vi "GDSFile_CreateFolders.vi"(1 "Path":path, 3 "Promt if folder\ndoes not exists?":bool=TRUE, 5 "error in (no error)":errorcluster) -> (13 "log error":errorcluster, 14 "PathOut":path, 15 "File permission error!":bool, 16 "Folder exists?":bool, 19 "error out":errorcluster)   [LabVIEW 2020]
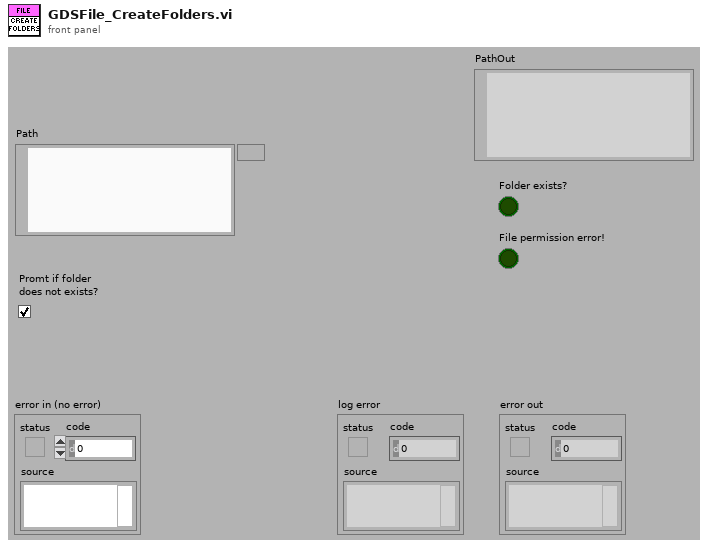
[diagram p1: front panel]
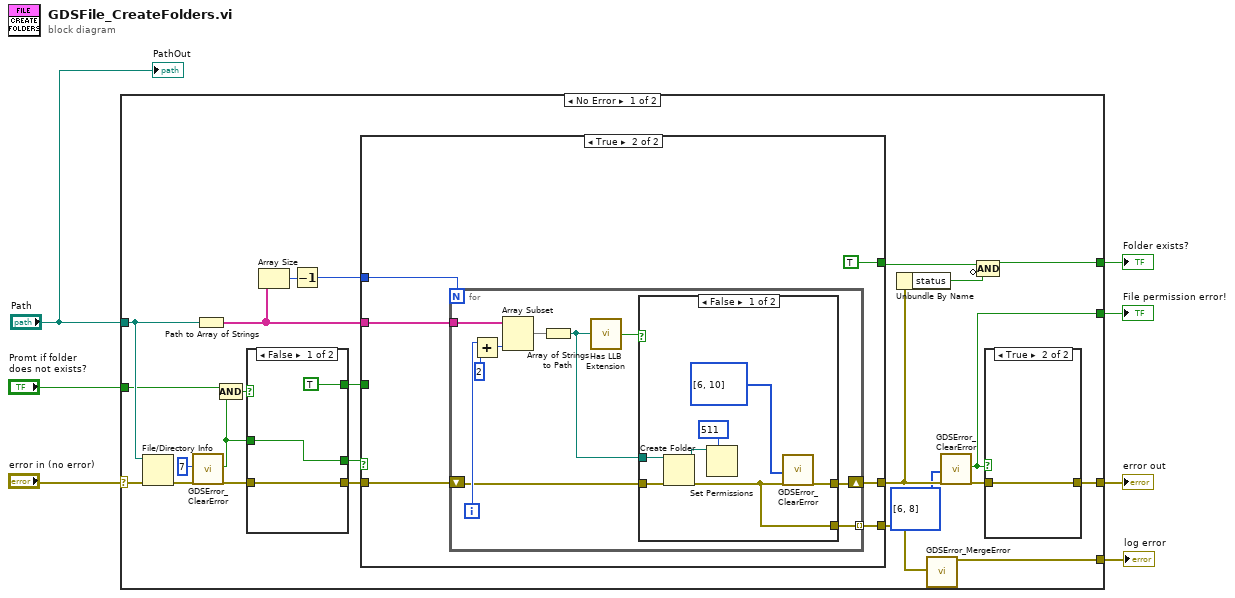
[diagram p0: block diagram]
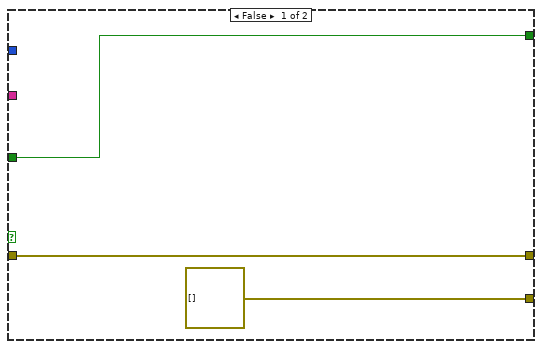
[diagram p3: hidden frame]
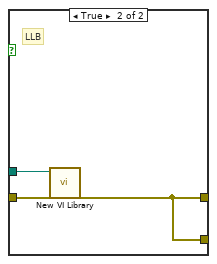
[diagram p4: hidden frame]
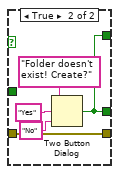
[diagram p5: hidden frame]
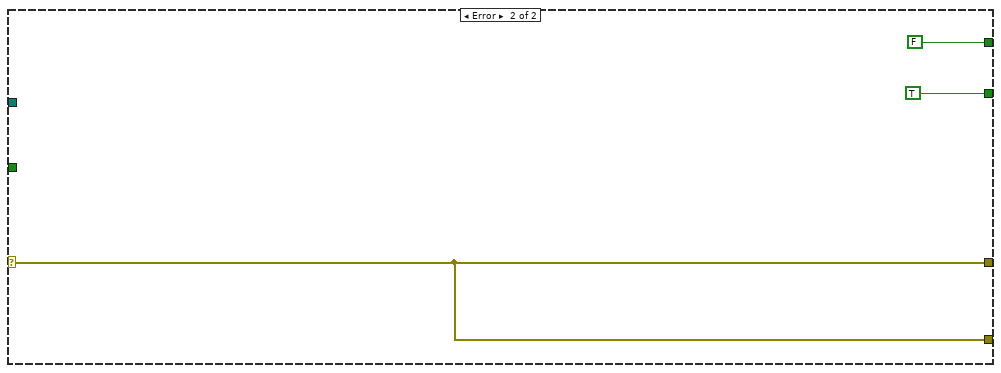
[diagram p6: hidden frame]
diagram:
  n1 = case shown="No Error" "error in (no error)" {
    selector: "error in (no error)" -> [w31 w71]
    tunnel: "Path" -> [w30 _]
    tunnel: [w23 w71] -> w6
    tunnel: [w22 TRUE ("Cleared?")] -> w5
    tunnel: [w18 FALSE] -> w4
    tunnel: "Promt if folder\ndoes not exists?" -> [w15 _]
    tunnel: [w9 w71] -> w2
    frame No Error {
      n2 = File/Directory Info(path=w30, error in=w31) -> (error out=w29:errorcluster)  [unwired: 6 out]
      n3 = call "GDSError_ClearError.vi"("code"=7, "error in (no error)"=w29) -> ("Cleared?"=w14:bool, "error out"=w27:errorcluster)  [unwired: 16 in]
      n4 = Path to Array of Strings(0:w30) -> (2:w13:string[])  [unwired: 1 out]
      n5 = Compound Arithmetic op=AND(w15, w14) -> (w16:bool)
      n6 = case shown="False" w16 {
        tunnel: w27 -> [w65 w67]
        tunnel: [w65 w67] -> w25
        tunnel: [w63 w66] -> w26
        tunnel: [TRUE w66] -> w17
        tunnel: w14 -> [w63 _]
        frame False {
        }
        frame True {
          n7 = Two Button Dialog(message="Folder doesn't exist! Create?", 1:"No" ("F button name (\"Cancel\")"), 2:"Yes" ("T button name (\"OK\")")) -> (T button?=w66:bool)
        }
      }
      n8 = Array Size(array=w13) -> (size(s)=w12:i32)
      n9 = Decrement(x=w12) -> (x-1=w11:i32)
      n10 = case shown="True" w26 {
        tunnel: w13 -> [_ w39]
        tunnel: [w36 w42] -> w21
        tunnel: w25 -> [w36 w40]
        tunnel: [w35 TRUE] -> w20
        tunnel: w17 -> [w35 _]
        tunnel: w11 -> [_ w38]
        tunnel: [errorcluster[] [] w37] -> w8
        frame False {
        }
        frame True {
          n11 = for {
            N: w38 -> [_]
            shift-right: [w44] -> w42
            shift-left: w40 -> [w46]
            tunnel: w39 -> [w52]
            tunnel: [w43] -> w37 mode=indexing
            i -> [w51]
            n12 = Add(x=w51, y=2) -> (x+y=w50:i32)
            n13 = Array Subset(array=w52, length=w50) -> (w48:string[])  [unwired: 1 in]
            n14 = Array of Strings to Path(0:w48) -> (2:w45:path)  [unwired: 1 in]
            n15 = call <vilib>:"Has LLB Extension.vi"("path"=w45) -> ("path to VI library?"=w47:bool)
            n16 = case shown="False" w47 {
              tunnel: w46 -> [w59 w62]
              tunnel: w45 -> [w58 w61]
              tunnel: [w57 w60] -> w44
              tunnel: [w55 w60] -> w43
              frame False {
                n17 = Create Folder(path (use dialog)=w58, error in=w59) -> (created path=w53:path, error out=w55:errorcluster)  [unwired: 1 in, 1 out]
                n18 = Set Permissions(7:i16 511 ("permissions"), 11:w53) -> ()  [unwired: 3 in, 2 out]
                n19 = call "GDSError_ClearError.vi"("codes"=i32[] [6, 10], "error in (no error)"=w55) -> ("error out"=w57:errorcluster)  [unwired: 16 in, 1 out]
              }
              frame True {
                # "LLB"
                n20 = call <vilib>:"New VI Library.vi"("error in (no error)"=w62, "VI library path in"=w61) -> ("error out"=w60:errorcluster)  [unwired: 8 in, 1 out]
              }
            }
          }
        }
      }
      n21 = Unbundle By Name(w21) -> ("status"=w19:bool)
      n22 = call "GDSError_MergeError.vi"("Error Array"=w8) -> ("error out"=w9:errorcluster)  [unwired: 17 in, 1 out]
      n23 = call "GDSError_ClearError.vi"("codes"=i32[] [6, 8], "error in (no error)"=w21) -> ("Cleared?"=w22:bool, "error out"=w24:errorcluster)  [unwired: 16 in]
      n24 = Compound Arithmetic op=AND(w20, invert w19) -> (w18:bool)
      n25 = case shown="True" w22 {
        tunnel: w24 -> [w32 w33]
        tunnel: [w32 w33] -> w23
        frame False {
        }
        frame True {
        }
      }
    }
    frame Error {
    }
  }
  "error out" <- w6
  "File permission error!" <- w5
  "Folder exists?" <- w4
  "log error" <- w2
  "PathOut" <- "Path"
